vi "Temperature Monitor.vi"() -> ()   [LabVIEW 2014]
doc: "This VI uses a While Loop and shift registers to average data. No hardware is necessary."
panel:
  in  "Stop Button":bool
  out "Temperature History":cluster{dbl, "Temperature Value":dbl}(graph)
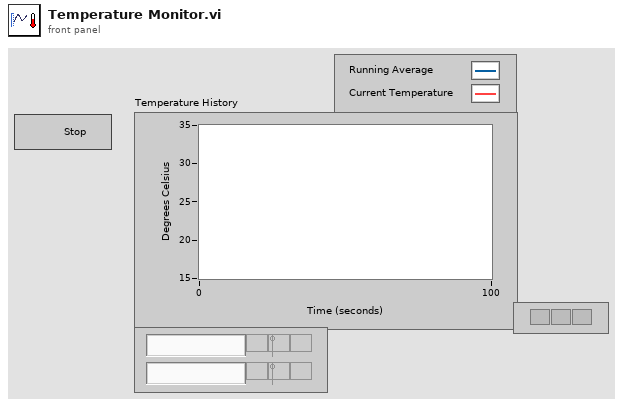
[diagram p1: front panel]
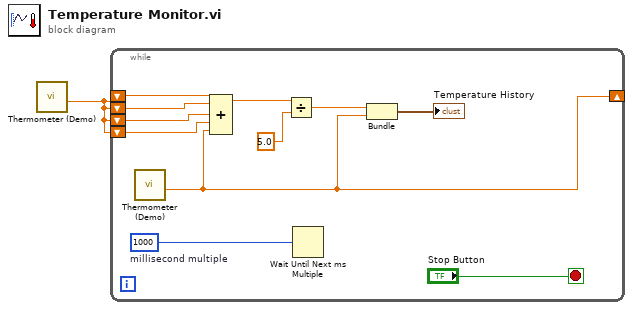
[diagram p0: block diagram]
diagram:
  n1 = call "Thermometer (Demo).vi"() -> ("Temperature Value"=w1:dbl)  [unwired: 11 in]
  n2 = while {
    shift-right: [w2] -> _
    shift-left: w1 -> [w11]
    shift-left: w1 -> [w10]
    shift-left: w1 -> [w7]
    shift-left: w1 -> [w6]
    stop <- "Stop Button" stop-if-true
    w12 = u32 1000  # millisecond multiple
    n3 = call "Thermometer (Demo).vi"() -> ("Temperature Value"=w2:dbl)  [unwired: 11 in]
    n4 = Compound Arithmetic op=ADD(w11, w10, w7, w6, w2) -> (w9:dbl)
    n5 = Divide(x=w9, y=5.0) -> (x/y=w4:dbl)
    n6 = Wait Until Next ms Multiple(millisecond multiple=w12) -> ()  [unwired: 1 out]
    n7 = Bundle(w4, "Temperature Value"=w2) -> (→"Temperature History":cluster{dbl, "Temperature Value":dbl})  [unwired: 1 in]
  }
